vi "Battery First Match Test Bench.vi"() -> ()   [LabVIEW 2014]
uses:
  Controls/PC Data.ctl
  Controls/MicroZed Config Op Mode.ctl
  Controls/ES String Array.ctl
  Controls/ES String Data.ctl
panel:
  in  "Boolean":bool
  out "DC Link Command":sgl
  out "Close Command Sent":bool=TRUE
  out "ES ON Array":bool[](array[boolean])
  out "Contactor Closed":bool=TRUE
  in  "ES String Data":T1
  in  "String Index":i32
  in  "PC Data":T3 {"Alarms 2" format="%016b"; "Faults 2" format="%016b"; "Alarms 1" format="%016b"; "Faults 1" format="%016b"; "Contactor FB" format="%.0b"; "Clear Faults SP" format="%.0b"}
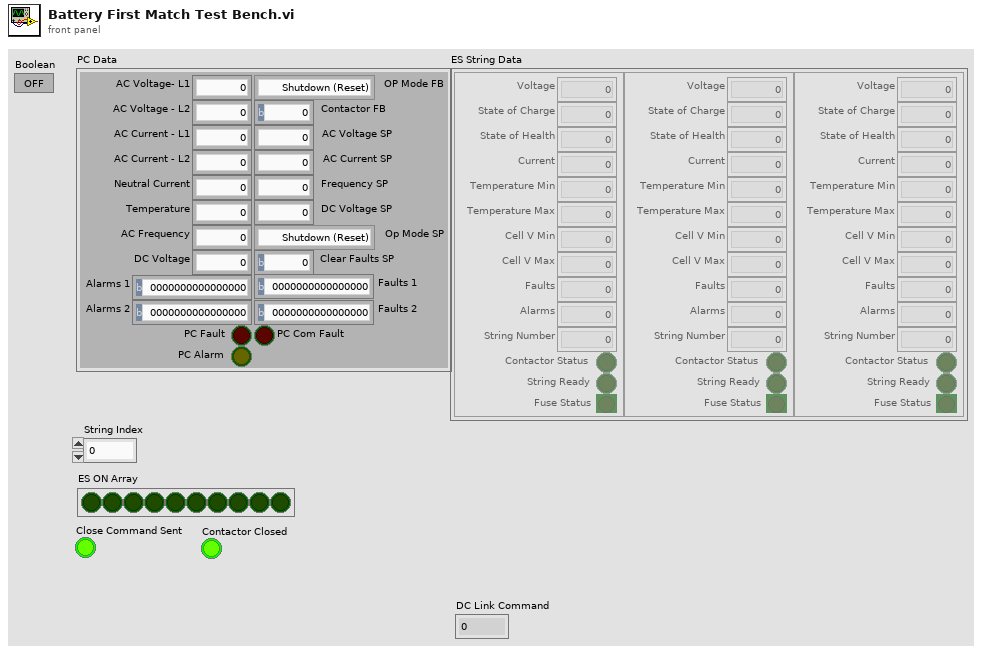
[diagram p1: front panel]
types:
  T1 = typedef "ES String Array.ctl" = T2[]
  T2 = typedef "ES String Data.ctl" = cluster{"Voltage":sgl, "State of Charge":sgl, "Current":sgl, "Temperature Min":i16, "Temperature Max":i16, "Faults":u16, "Alarms":u16, "String Number":u16, "Contactor Status":bool, "String Ready":bool, "Fuse Status":bool, "Cell V Max":dbl, "Cell V Min":dbl, "State of Health":sgl}
  T3 = typedef "PC Data.ctl" = cluster{"AC Voltage- L1":dbl, "AC Voltage - L2":dbl, "AC Current - L1":dbl, "AC Current - L2":dbl, "Neutral Current":dbl, "Temperature":dbl, "AC Frequency":dbl, "DC Voltage":dbl, "AC Voltage SP":dbl, "AC Current SP":dbl, "Frequency SP":dbl, "Op Mode SP":T4, "Clear Faults SP":u16, "PC Com Fault":bool, "PC Fault":bool, "DC Voltage SP":dbl, "OP Mode FB":T4, "Contactor FB":u16, "Faults 1":u16, "Alarms 1":u16, "Faults 2":u16, "Alarms 2":u16, "PC Alarm":bool}
  T4 = typedef "MicroZed Config Op Mode.ctl" = enum16{"Shutdown (Reset)", "Startup", "Idle", "Voltage Mode", "Current Mode", "Fault", "OL Voltage (Debug)"}
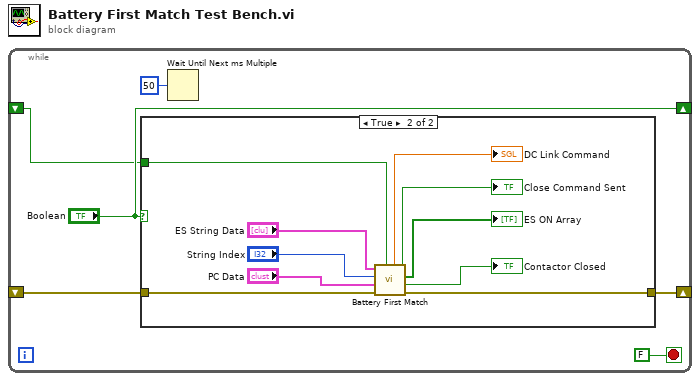
[diagram p0: block diagram]
diagram:
  n1 = while {
    shift-right: [w4] -> _
    shift-left: _ -> [w3]
    shift-right: ["Boolean"] -> _
    shift-left: _ -> [w1]
    stop <- FALSE stop-if-true
    n2 = case shown="True" "Boolean" {
      tunnel: [w7 w10] -> w4
      tunnel: w3 -> [w7 w9]
      tunnel: w1 -> [_ w8]
      frame False {
      }
      frame True {
        n3 = call "Battery First Match.vi"("Safety Init"=w8, "Error In"=w9, "PC Data"="PC Data", "String Index"="String Index", "ES String Data"="ES String Data") -> ("Error Out"=w10:errorcluster, "Contactor Closed"=→"Contactor Closed":bool, "ES ON Array"=→"ES ON Array":bool[], "Close Command Sent"=→"Close Command Sent":bool, "DC Link Command"=→"DC Link Command":sgl)  [unwired: 2 in]
      }
    }
    n4 = Wait Until Next ms Multiple(millisecond multiple=u32 50) -> ()  [unwired: 1 out]
  }
